vi "2023_day14_Task1.vi"() -> ()   [LabVIEW 2021]
uses:
  <userlib>/_OpenG.lib/array/array.llb/Search 1D Array (String)__ogtk.vi
panel:
  out "Task 1":i32
  in  "Switch":bool caption="Ex. Data  vs.  User Data"
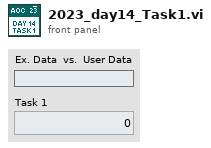
[diagram p1: front panel]
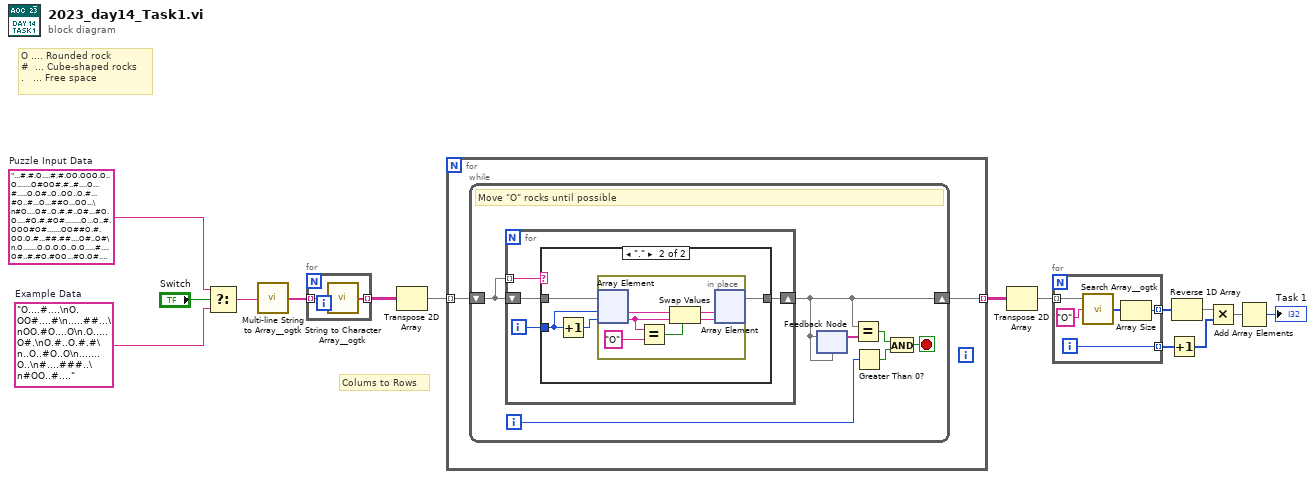
[diagram p0: block diagram]
diagram:
  w13 = "...#.#.O....#.#.OO.OOO.O..O.......O#OO#.#..#....O...#.....O.O#..O..OO..O.#...#O..#...O...##O...OO...\n#O....O#..O.#.#..O#...#O.O....#O.#.#O#........O...O..#.OOO#O#.......OO##O.#.OO.O.#...##.##....O#..O#\n.O.......O.O.O.O..O.O.....#....O#..#.#O.#OO...#O.O#.O#..#O...#...O.O.......#.O....O.#..#.O##O#..O...\n...O....#.OO..#..OO#..##....#O.......OOOOOO...OO..#...#.O..O....#O..OO.#O...#O#...O..O#..OO....#....\n..O...##OOO....#..OO.OO#O##..#.#........O#.#.....#OO...#............#.###..#.#O...#..O.#O#.O#O.....#\n...............O.....##..O...O#.O#........#.O.#..#...#..O..O.#...#......#......O.OO.OOO.#.O.....O##.\n......#..#..###.OO.#......O..O.O##O..O.....OO.#.OO....O.....OO#O..O....#.....#.#.O#..O..O.OO.O#O.O.#\n##O.....O.#.#O...#.#O###....#.O#.#..#..O.#O........O.OO..#..#O#.O#..OO..#.O.##O....#.##O.O.......##.\nO#...###...O..#...#......O#.OO.....#...OOO...#.#O.#...##..OO#.......#OO.....#...O...#.#O.........O.O\n..O....O....OO..O.O.O........#.O#..O.#..#..OO#.OO..#.O...O..#...O..##..O........O##..........OOO..OO\n....##......#.#.O.O#O##.#....#..O#............#..#...#......#O.OO#....O.......O###....O...........OO\n.O.OOO..O#....O...O..#.O#.#O.O...#.O..O#...OO#.#....#OO.#........#O.......O...#O......O...O....#...#\n.#....#O...##..#.#..........O..#O........OOO.......O.OO.##...#..........#......#.O##.#O#OO#OO..#..O.\n......#O...#.#.......O........#O....#O..##....O......O.#.O..#OO............O##O....#O.OO#..O#..O#...\n..OO.....O#O..#OOOO#O.##.........O..#OO#......O.OO.....O......OO..O...O..O....O..O#O.......O..O.O#..\n....O...OO....##.....OOO...O#O.#.O...O.....#........#.#O#.....O.O.OO.###.#.OO#OO....O.....O..#.#O...\n.OO#..O#O#O...#..O.O....O#.O.#........O.O..O....#O#....#.#.O#.#...O.O..O..#..#...OO#O......#O.O..O.#\nOO...O.O.#..#....#...#O.O##O#...#............##.O..OOO....O..OO....#OO....O.#....O#.O........OO..#..\n..O#.OO#.#O#..O.......O.##.O.#....OO#.#O#.##.O..O#..####....#..#......#...##.O##...O....O..#.#......\n#O.O#.....#....O...O.O..O.O.O#O.O#....#..O...#.O.#O...#..#.#O.....#O..##...O.......O.....O..OO#OO##.\n..O.#..#...O....#.##.#.O......#.#.##.......#.O..##O#.#O.OOO..O...#O......#..O.....O.OO...O#.O.#OO#.O\n.#..OO#.......OO....O.##...O......O.OO#.O......#O..O#..#..O.O..O.#..OO.O.#O..O..#......O...O....O#..\nO....#.#O..O#...#..##..##.O.O.O..O.O#...O#..#O.O......#O.......O..O.O...#.#O..OO#.#.....#O#...O..#.O\n...O...O.O.O.OO..O....O..O..O##..O.........O#O..O.#...#.O..O.#........#...O........O#.#.O..O.....#..\nOO....O#...........#OO......O.....O...#...OO....OO..O.........O.#......##O....#...O##....O.#...#...#\n#OO#....#......OO.O....O...#..O...#.OOOO..OOO.O.O...O#.......O....#O#O.O#O......#...#...OO#.O...#..#\n....O#.#...O..#.................#.#...O...O...O.O#.##..O.#.#....####..OO....O.......#.OO.O....#...#.\n.....O.#.#O..#O...#OO....OO...O#..O...O..#O..O....#.#O..#.......O...O.O.....#.##.#O.OO..#.#....###..\n.#O..#...#...#.#.O.#O.#OO..#.#..#O#.#.#O#.O#O#..##..#...#O#.#..#.OO#..#..#..O...O...O..O...#.O....O.\n..O.....#....#O#OO#O.....O.....O...OO.O......OO..O....O...#....O....#...OO....O..O...#...###O.....#.\n##..##...#OOO...#.OO...#.#.O#.O.........O.O.#.O..O.OO#.O......#.###...#..#O.#....#...#.O..##...#O...\n.O.#...O.O....O.......O...#O.....O......OO..OOO##.#...##OO.O......#....O..#..#.##.OO.......#O...#OO.\n...#...O#..O.#.OO.#.OO..O.#O.#.O.#...O#....O#.O#......OO.#....#..#..#..#....O.#....##...............\n.O.O#....#.#.....O...#.O#O#.......#.#O..OO.O...#....#.....O.#.#.#..#...#...##..O.O...#O..O.#..#O....\n.#......O..O#...O.O.##O..#.OOOO.O#O....O#...#O..OO.#.#O......#..O..O.OO#OOO#O#.O.......OO.....O...#O\nO##.O..OOO.#..O......#...#O#.O.O#..O.OO..#......O.O.O..O.O.OO..#....O.#O...O#.#..#..O.#...##O.O.....\n.#OO#....#.....#..OO.OO...##.O......OOO.#O..O#.O.O.........O#.O.#.#...#..##...#O.O..OO.O#.#..O..O.O.\n.O.....#.O#....O#.....#.O..O..O#..#..OOO#O....#OOOOO.#.#.........O#..O.#....#.#....O.#..##..#.......\n..O.#OO....#O.#...#O...#.O#..#.O....O.#..O....O#.....O.OO..OO.OO#.#..#..#O.O.#...O....OO...O.#..O..O\n.O.OO#...O#.OO....#.O....O.###...#..O.....O....#.O..O.#O.O.....#....#O#O...#..O...O........O...#....\n#...#...#..O..#.##.#.....O#..#O.##.O...O...#....O.O.O..O.O........O.O.O.....O..#.......#...O..O.#.#O\n#O...#...O.#....#.O.....OOO..O...OO#OO#.......#O.##...#.O#O#....#.....O#..OO.#.#.O.O..O.#OO.O.#..O..\n......O.......O.#.O.#.O...........O.O.OO#....#OO........O#.......OO.O..#O...#....O#..O....OO..O##...\n.##..O..#O...O.O....#O#..OO#O.#....#O.OO#O....#.....#...#.#OO#.OO.#.O.O.O.OO.#O.O.#.O....#O.O.O..O..\nO#..O#O##.O....O..#......O....#..O##O.O#...O...O...OO#..#OO...O##.#....O#.O..O.......#..#......#O..#\nO.OO..O..#.O..O#OO#O.....#O..O..#...#.OO.O..O...........O...O...OO##.#..O..#.#.OO.#.#...O.O......O.O\n.O.O##.O....#O.O...O#.#..O....#O.....O..O#OO....OO##.#.O..#O.O...O..O.O...#O.OO.........#.##OO#..#..\n..OO....O.....#....O.....O...OOO#...#.O.........O.O..OOO.###O.#.......#.#...O.OO.#..O.....#O.....#..\nO...##O...O..##..#.#...#.#O#.O...#.#.O..O....##......#...#.O..O...OO.#...OOO#OO...O.O#O..OO.O##O..O.\n..#.OO.#.##..O....#...OO.#O.......O.O#...O..#.#O..O.###O#.#.O.O...O.#O.#..#.O..O#O#..O.........#.#..\nO.#.O##.......OO#....O#.......O..O.....#.........O.O.....#O.......#O..#.O...#....O.#....#......O.O.#\n.OO.O...O.......#O#....#O#...#.........O..O.#.OO#.OO.O#...#O...O..#..O##O.#...O#..O.OO.O...#OO.##.#.\n...O.O...OOO.O......#..O...#.##.O..O..#...O.O...#.O.O..OO..OO..#....O.O#..#...O.OO.#.....#...OO#...#\n.#............#O.OO..O#.....O..#O.#O.##O....O.O....O..O#..O..O.#..O.#.O.#.O.#..#O.#.OO.O......##...O\n#.....O.#..O.O........O#O#OO..OO.....#.#....OO##......O.O.##..##.#.O...O.#.#O......O..##.#.#.#..#O..\n##.#.O..O...O..OO...O....O.O..O#...OO....OO#.#...#.#....OO#..........O..O...O...O........#..O##.#.#.\n..OO.#..#.OO..#O..#.O...OO.O...O....#..OO....#OO..#........#...O..........#..O...OO.O.......#.#..##.\n.#.#...#O.O.#.O..O.OO.OO#..OO#OOO#O....O..O#..OO.O..##..#.#....OOOOO#....OO..O....#..O..............\n...O#.OO......O.#.O.#.#O.OOO...#OO..#....#.O.O.O.......#...##...O...OOO..##...O....O...O.#...O.O...O\n..O...O..#.O.....#.#..##.......####...##.......O...O#.##....O.#..OO....#.#.O...##O.#O.###.OO#....O.O\n.O#..#....OO...O.O.......O#OO..O#.O.O..#......#..O.#..#O......OO.O...O.....O........O#.#O.#.#.##.O#.\n..O....O.#...#..##..O...#.O#..OO...O.......#OOO......#O..OO...O...#..O...##O.#...#.#.##...O...#.OO..\nO.#..#...O#OO.O#.O..O.....O.O..#.#.##....O.O..O......OO.O.#.....#....#.##...#...O..O........#......#\n.OO.OO.........#...#.#O...#..#..#.###O....#...OO#......#O.O..........#O...#.#.#O#..........#.O#...OO\n##.#..#O#OO.#.....O......#....O..#.O#..#.OO.........#.......#.#..#..O.O#OO.###.O.#.#O..##....O.O..O#\n#...O...O.......O#.O.#..#O#.O...O...O...O.O.#.O....O###..#.O..O.....O..OO#...O.#...#....O.#O..OO.O..\n#O...O...O.##..#.#OO.....#O.#..O....#O.O....O.....#.O.....#.O.O....#.......O.#.O..#.O.##....O..O..O#\nO..O.....#O..O...O........O..#.#..........##O#..#..O.#.#OOO..#..O...O..O..#.O....O...O...#...#...O..\n#...O.......O#..#.O#.O.....#....O#O......O..O.....#.....O...#...O...#O..#.O..#..#....O....##O#.....#\nO...O..#O#.OO..##..#.......O.........#......#...#..O.O..#..#O..O..O.OO......O#OO.#..O#....#.O.#.....\n.....#.OOO..OOO....O...#O....O.#.O.#.#O..#O.......O#..O.#O.#.#..#......O#O###..#.#.O..OO.O#.##.OO#.#\nO...#..O#.##O..#...#.....O...O.O............O#.....#.O....O#....O#.#O#O..O#.OO..........#.O.#OOO.O..\n......#..#...O..O....OO#.O...OO..O....O..##O#..O#..O..##.O..#....##OO.....#..O#.O....#O.#....##.O...\n.#..O.O..#..........O...O...O.#..O.#......O.O.....OO#..#...O.....O##..O.O..#.OO.#O.O....O...O..#..#.\n.OO.#..O......#........#.#.O...#..........O..O.O.......OO..##O.....#...O...#..#O###..O..O.OOOOO.#.O.\n.O..#..O..O...O..#O......OOO.O#..O#.#O...O#O.#...O....O..OO.#....#...O#................O.#O..O.#O..#\n......O..O...##..O..##.O.####..OO.O.......#.#O..O#..O#O.......#..O.....##........#..O..O.#...O....OO\n.....O.O.O.....O..OO..#O..O#.#OO....#O...#O#.#.OO.#..O...O.#.....#.#O#..O#...OO##.........##...##..#\n....O..OOOO..O.O...#.....#.#..OOO...#OO.O#..O..O....#O.......#.O..OOO......OO...#.O#............O#.O\n......O....#...#.#..O.O#.#...O..O.OO##.O..O#OO##...#.#..O.OO.........#..##O#...O.#..O.#OO.#O#...##O.\nO..##.O...O..#.O.O.O..O.........#..O...#..O.O.##O#.O..#.#.....#..#O#..#.OOO#.O..O...OO#.O...O#......\n.O.....O......O.......O#..O.OOOO..O..OO.O#.##.OO#O#.O......#...#.........O..O#...#O..#..#.O...O.#OO.\n#O.O...#..OO.#...O.O#....#..#...#OOO##.O.OO#.....#.O#.O..O.#O#O.O.O..........O#.O#.#O###O..#..#.#OO#\n#O###.O..O..O......#.O#.#....OO..O.O#....#...#...#.##...OO..O.#OO........O....O..O....OO......O..O.#\n.O#O..O...#OOO...O.O...#.O#......#......#O.....O.#.#.O.#....O#.#O..#...#..#...OO#.....OOO....OO.....\n..O.#.O....OO......O...O..##.O........#.O.#O.#...O...O.#.##OO.#O......O...O..O.O.O.##..O#.##.#.#O...\n.#OO#.#.O#O....O.O....OO#....##.....#.##O..O...OO.....#..O.#....O#.......O....OO.OOO.#...#..O.O.#.OO\n.O...O....#.O..O.#..#.........O.#O#.#...O..#O.O.O..O##.....OO..O.O..OO..O..#..#.#.O..#O..O.OO##....O\n.##...#O.O..OO..O..#.#O.O.OO.#..#.OOOO.....O...O.O.O#...O#.#.O.............O..O...#.#..........OO#.#\n.#....##O....##O..#.O.O..#..O##....#.#.OO........O.O#..#........#OO........O...#.OO..#.........#....\n.##OO..#O.#.O..OO.#...#O#.....O....O.#....#O..O#O.#.O..##.O.O.....#.#...#.O..OO....O....#.#.#.......\nO.O.O.#....#.OO.#...#...O..#.OO..#..O..#...O.OO.O...##...OO.O#O..O.OO.O##.....#..O#..#O....O.O#OO.#.\n.#.O....#.#....#..O.O....OO......O......O.#...O...#.O.O..#.#.....O..#O.O.O..OOO#.O#..O...O#..OO.....\n#.#O..#....#.....O.#....#......O.O..O.O.OO.O#...O.#.O.O...#....O...#..#...O.#.O..#.O...OO.#.#O###.OO\n..#..O..#O##..#.....O...#..O...OO..#.#.O.#.O.O.....O..O#O#..O......#...#O.O.OO..O............#....#.\n....O#....O#O###O.O..#.#..O.#.O.#.O....O........#O.OOO......O.OO....O.O.O.....##.O#....##O.#.OO..O.#\n..#.O...OO.#O.#..OO.##..#...O#..O#..#O.O..#......O.....##....O...O.O#OO#O.......O##OOO.OO.O...O.#..#\nO......#.O.....OO.OO.O...O.#O..O...O.#.#...#...O...#.OO.O.#.#OO.....#.O.#....OOO........##...##.##O.\n#O...#....#...##O.#......O#...#O..........##O..#.O.#O#..#...OO.O....O..##..#...#...#..O..O....O..O#.\n...OO....O#..O..#....O.#.#.....OO.#..#O..OO.#.#.#.#......O...O..#.#..##.....#...O.##.....O#.#..O#O.."  # Puzzle Input Data
  w14 = "O....#....\nO.OO#....#\n.....##...\nOO.#O....O\n.O.....O#.\nO.#..O.#.#\n..O..#O..O\n.......O..\n#....###..\n#OO..#...."  # Example Data
  # "Colums to Rows"
  # "O .... Rounded rock\n#  ... Cube-shaped rocks \n.   ... Free space"
  n1 = Select(t=w13, s="Switch", f=w14) -> (s? t:f=w12:string)
  n2 = call <userlib>:"Multi-line String to Array__ogtk.vi"("string"=w12) -> ("lines"=w11:string[])
  n3 = for {
    tunnel: w11 -> [w17] mode=indexing
    tunnel: [w16] -> w9 mode=indexing
    n4 = call <userlib>:"String to Character Array__ogtk.vi"("Input String"=w17) -> ("Character Array"=w16:string[])
  }
  n5 = Transpose 2D Array(2D array=w9) -> (transposed array=w10:string[][])
  n6 = for {
    tunnel: w10 -> [w19] mode=indexing
    tunnel: [w18] -> w6 mode=indexing
    n7 = while {
      shift-right: [w24] -> w18
      shift-left: w19 -> [w26]
      i -> [w23]
      stop <- w20 stop-if-true
      # "Move \"O\" rocks until possible"
      n8 = for {
        tunnel: w26 -> [w30] mode=indexing
        shift-right: [w27] -> w24
        shift-left: w26 -> [w28]
        i -> [w29]
        n9 = case shown="\".\"" w30 {
          tunnel: [w31 w33] -> w27
          tunnel: w29 -> [_ w34]
          tunnel: w28 -> [w31 w35]
          frame Default {
          }
          frame "." {
            n10 = Increment(x=w34) -> (x+1=w32:i32)
            n11 = in-place {
              n12 = in-place-array #1(w35, w34, w32) -> (w39:string, w38:string)
              n13 = Equal?(x=w38, y="O") -> (x = y?=w40:bool)
              n14 = Swap Values(12:w39, 13:w40, 14:w38) -> (1:w36:string, 3:w37:string)
              n15 = in-place-array #1(w36, w37) -> (w33:string[])  [unwired: 2 out]
            }
          }
        }
      }
      n16 = feedback-in #2(w24) -> ()
      n17 = feedback #2(w24) -> (w25:string[])
      n18 = Equal?(x=w24, y=w25) -> (x = y?=w21:bool)
      n19 = Greater Than 0?(x=w23) -> (x > 0?=w22:bool)
      n20 = And(x=w21, y=w22) -> (x .and. y?=w20:bool)
    }
  }
  n21 = Transpose 2D Array(2D array=w6) -> (transposed array=w5:string[][])
  n22 = for {
    tunnel: w5 -> [w44] mode=indexing
    tunnel: [w43] -> w4 mode=indexing
    tunnel: [w42] -> w1 mode=indexing
    i -> [w42]
    n23 = call-poly <userlib>:"Search Array__ogtk.vi"("Array"=w44, "Element Data"="O") -> ("Indices of Elements"=w46:i32[])  [unwired: 7 in]
    n24 = Array Size(array=w46) -> (size(s)=w43:i32)
  }
  n25 = Increment(x=w1) -> (x+1=w8:i32[])
  n26 = Reverse 1D Array(array=w4) -> (reversed array=w2:i32[])
  n27 = Multiply(x=w2, y=w8) -> (x*y=w7:i32[])
  n28 = Add Array Elements(numeric array=w7) -> (sum=→"Task 1":i32)
